vi "StartStreaming.vi"(8 "error in (no error)":errorcluster, 11 "CameraDemo in":refnum<class "CameraDemo.lvclass">) -> (0 "error out":errorcluster, 3 "CameraDemo out":refnum<class "CameraDemo.lvclass">)   [LabVIEW 2020, in "CameraI2COUSB.lvlib" / "CameraDemo.lvclass"]
doc: "Start streaming"
uses:
  CameraDemo.lvclass
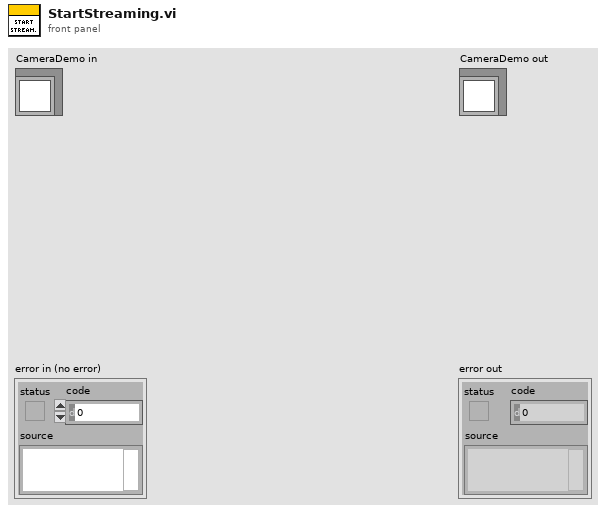
[diagram p1: front panel]
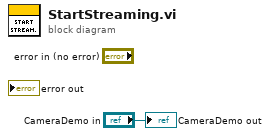
[diagram p0: block diagram]
diagram:
  "CameraDemo out" <- "CameraDemo in"
